vi "SSH_Write.vi"(8 "error in (no error)":errorcluster, 10 "Text to write":string, 11 "Python":T1) -> (0 "error out":errorcluster, 3 "Python":T1)   [LabVIEW 2021]
uses:
  PythonCtrl.ctl
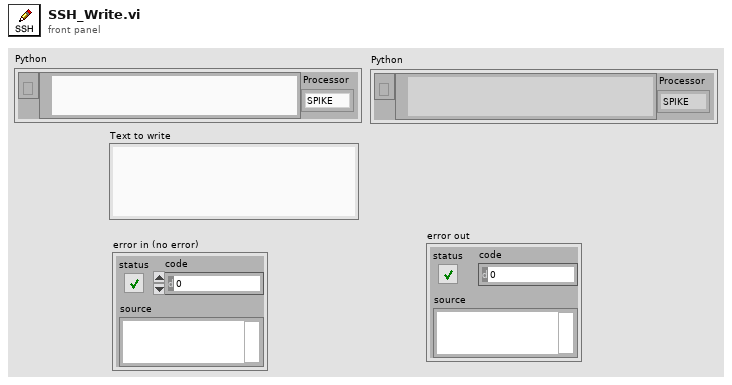
[diagram p1: front panel]
types:
  T1 = typedef "PythonCtrl.ctl" = cluster{"session":refnum<k35>, "PyPath":path, "Processor":enum16{"SPIKE", "Pi", "Pi_ssh"}}
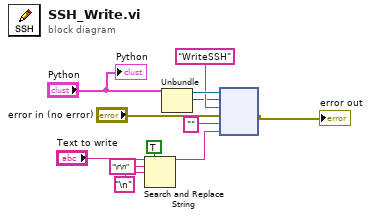
[diagram p0: block diagram]
diagram:
  n1 = Search and Replace String(replace all?=TRUE ("replace all? (F)"), input string="Text to write", search string="\r\n", replace string="\n" ("search string")) -> (result string=w11:string)  [unwired: 4 in, 3 out]
  n2 = Unbundle("Python") -> ("session"=w12:refnum<k35>, "PyPath"=w2:path)  [unwired: 1 out]
  n3 = node(w12, w2, "WriteSSH" ("function name"), "error in (no error)", "" ("function name"), w11) -> (→"error out":errorcluster)  [unwired: 2 in, 3 out]
  "Python" <- "Python"
